vi "TCam_WellTemp.vi"(8 "Well Pos":T2[](array[typedef]) {"Y" format="%.2f"; "X" format="%.2f"}, 10 "Pixels":cluster{"X":i32, "Y":i32}[][](array[cluster]), 11 "Image in":T1) -> (2 "Image Out":T1, 3 "Array":dbl[](array[numeric]))   [LabVIEW 2020]
uses:
  <vilib>/vision/Image Controls.llb/IMAQ Image.ctl
  <vilib>/Analysis/baseanly.llb/Mean (DBL).vi
  <vilib>/vision/NI_Vision_Development_Module.lvlib
  <vilib>/Analysis/NI_AALBase.lvlib
panel:
  out "x-y":u64
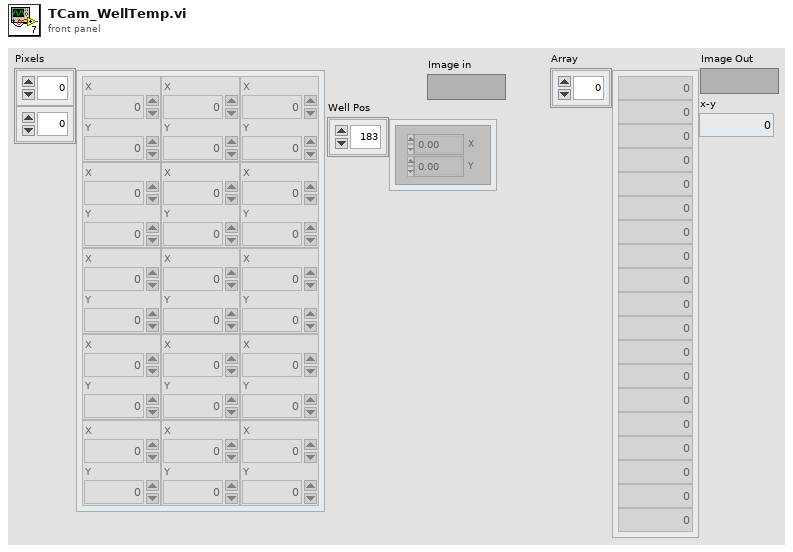
[diagram p1: front panel]
types:
  T1 = typedef "IMAQ Image.ctl" = refnum<image>
  T2 = typedef "IMAQ Point" = cluster{"X":sgl, "Y":sgl}
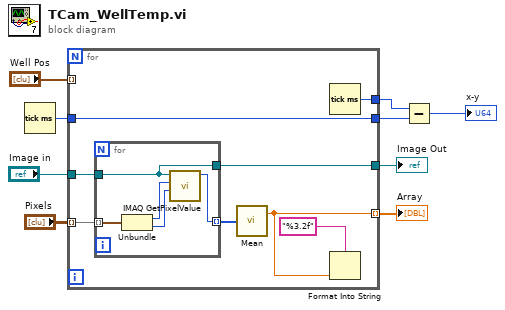
[diagram p0: block diagram]
diagram:
  n1 = Tick Count (ms)() -> (millisecond timer value=w4:u32)
  n2 = for {
    tunnel: "Image in" -> [w17]
    tunnel: "Pixels" -> [w16] mode=indexing
    tunnel: [w13] -> w8 mode=indexing
    tunnel: "Well Pos" -> [_] mode=indexing
    tunnel: [w14] -> w5
    tunnel: [w11] -> w3
    tunnel: w4 -> [w11]
    tunnel: [w10] -> w1
    n3 = for {
      tunnel: w17 -> [w18]
      tunnel: w16 -> [w22] mode=indexing
      tunnel: [w19] -> w15 mode=indexing
      tunnel: [w18] -> w14
      n4 = Unbundle(w22) -> ("X"=w21:i32, "Y"=w20:i32)
      n5 = call "IMAQ GetPixelValue"("Image"=w18, "X Coordinate"=w21, "Y Coordinate"=w20) -> ("Pixel Value (U8)"=w19:u8)  [unwired: 3 in, 4 out]
    }
    n6 = call-poly <vilib>:"Mean.vi"("X"=w15) -> ("mean"=w13:dbl)  [unwired: 1 out]
    n7 = Tick Count (ms)() -> (millisecond timer value=w10:u32)
    n8 = Format Into String(format string="%3.2f", w13) -> ()  [unwired: 2 in, 2 out]
  }
  "Array" <- w8
  "Image Out" <- w5
  n9 = Subtract(x=w1, y=w3) -> (x-y=→"x-y":u32)
